vi "Check Object Lengths.vi"(8 "error in":errorcluster, 11 "objects in":T1[](array[typedef]) {"Object ID" format="%x"}) -> (0 "error out":errorcluster, 3 "objects out":T1[](array[typedef]) {"Object ID" format="%x"})   [LabVIEW 2012, in "Device Data Model.lvclass"]
doc: "Checks to ensure that all Modbus objects can fit within the length allowed by the Modbus protocol data unit and will throw an error if any object is longer than allowed. This check must be performed because objects may not be split across multiple data units, although a request for multiple objects can be split across multiple responses."
uses:
  Device Data Model.lvclass
  Identification Parameters.ctl
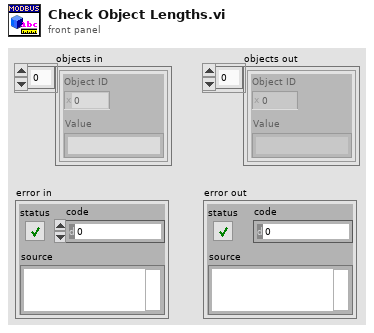
[diagram p1: front panel]
types:
  T1 = typedef "Device Data Model.lvclass/Identification Parameters.ctl" = cluster{"Object ID":u8, "Value":string}
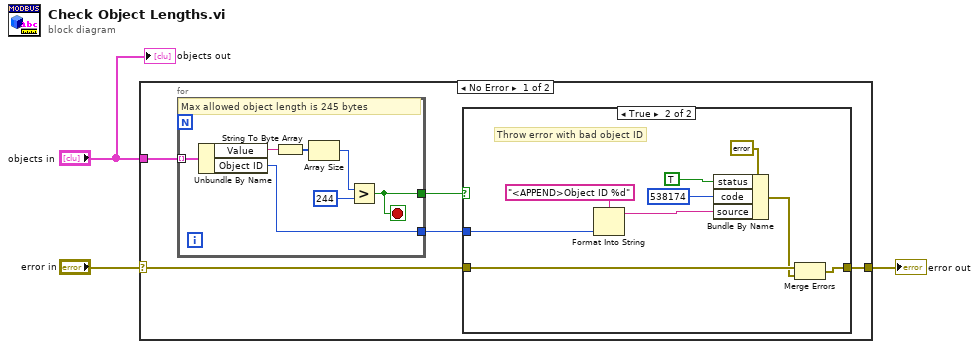
[diagram p0: block diagram]
diagram:
  n1 = case shown="No Error" "error in" {
    selector: "error in" -> [w6 w26]
    tunnel: [w5 w26] -> w2
    tunnel: "objects in" -> [w8 _]
    frame No Error {
      n2 = for {
        tunnel: w8 -> [w25] mode=indexing
        tunnel: [w20] -> w7
        tunnel: [w19] -> w4
        stop <- w20 stop-if-true
        # "Max allowed object length is 245 bytes"
        n3 = Unbundle By Name(w25) -> ("Value"=w24:string, "Object ID"=w19:u8)
        n4 = String To Byte Array(string=w24) -> (unsigned byte array=w23:u8[])
        n5 = Array Size(array=w23) -> (size(s)=w22:i32)
        n6 = Greater?(x=w22, y=244) -> (0:w20:bool)
      }
      n7 = case shown="True" w7 {
        tunnel: w6 -> [w9 w16]
        tunnel: [w9 w15] -> w5
        tunnel: w4 -> [_ w18]
        frame False {
        }
        frame True {
          # "Throw error with bad object ID"
          n8 = Format Into String(format string="<APPEND>Object ID %d", w18) -> (resulting string=w12:string)  [unwired: 2 in, 1 out]
          n9 = Bundle By Name(cluster=errorcluster {"status"=FALSE, "code"=0, "source"=""} ("error constant"), "status"=TRUE, "code"=538174 ("error code (0)"), "source"=w12) -> (w11:errorcluster)
          n10 = Merge Errors(w16, w11) -> (w15:errorcluster)
        }
      }
    }
    frame Error {
    }
  }
  "error out" <- w2
  "objects out" <- "objects in"
